vi "Dane.vi"(8 "error in":errorcluster, 9 "Ilość":string, 10 "PIN":string, 11 "Enum":T1(ring)=enum."Deposit") -> (0 "error out":errorcluster, 2 "Konto istniejące":bool=TRUE, 3 "Konto":T2)   [LabVIEW 2021]
doc: "Check if account exist\nReturn info account, account number, first name, last name, amount \nDeposit money and update file.\nWithdraw money and update file"
uses:
  Konto.ctl
  <vilib>/Utility/file.llb/Read Delimited Spreadsheet (string).vi
  <vilib>/Utility/file.llb/Write Delimited Spreadsheet (string).vi
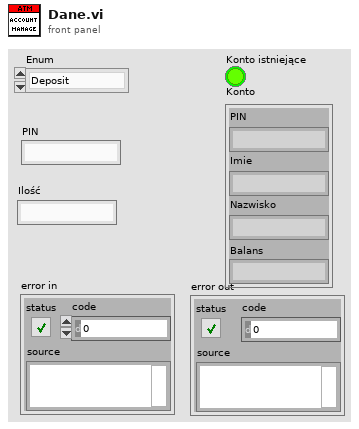
[diagram p1: front panel]
types:
  T1 = enum16{"CheckAccountNumber", "ReturnInfo", "Deposit", "Withdraw"}
  T2 = typedef "Konto.ctl" = cluster{"PIN":string, "Imie":string, "Nazwisko":string, "Balans":string}
  T3 = cluster{"all rows[0]":string, "all rows[1]":string, "all rows[2]":string, "all rows[3]":string}
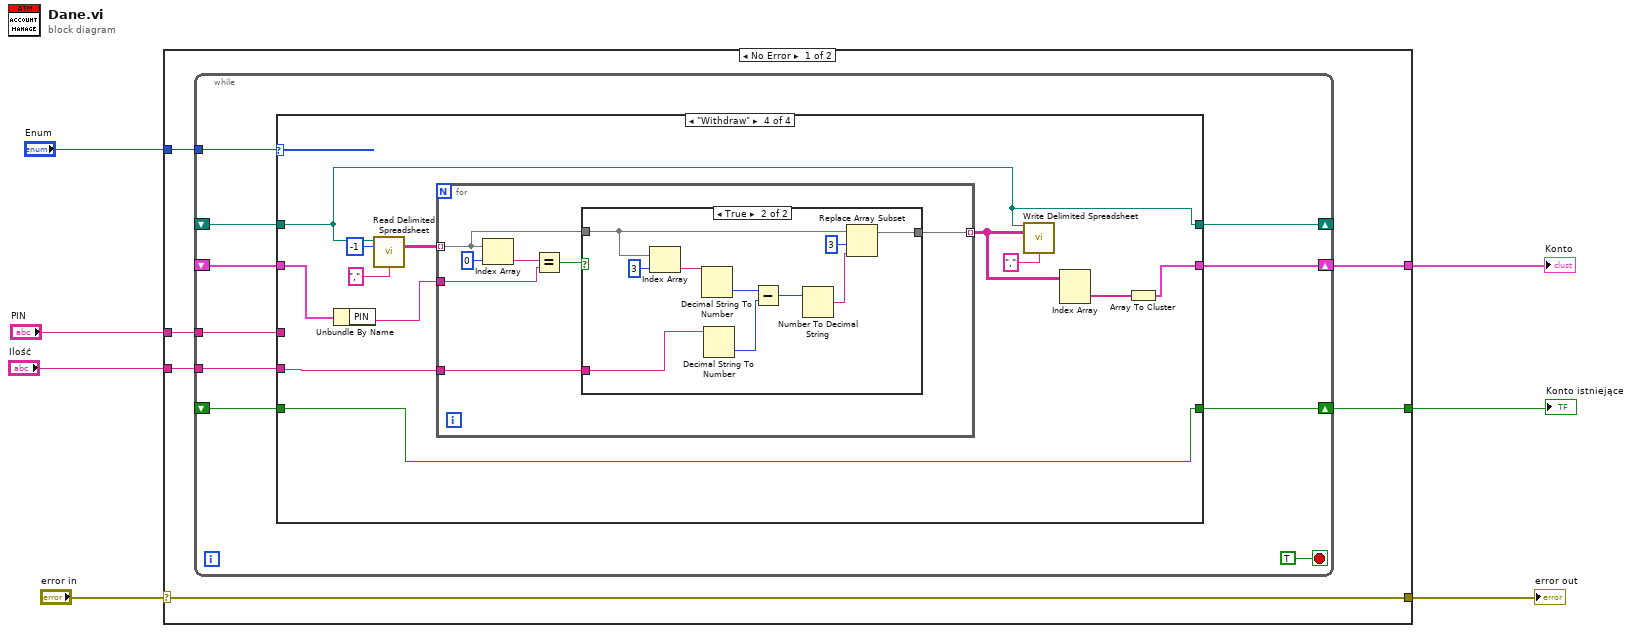
[diagram p0: block diagram]
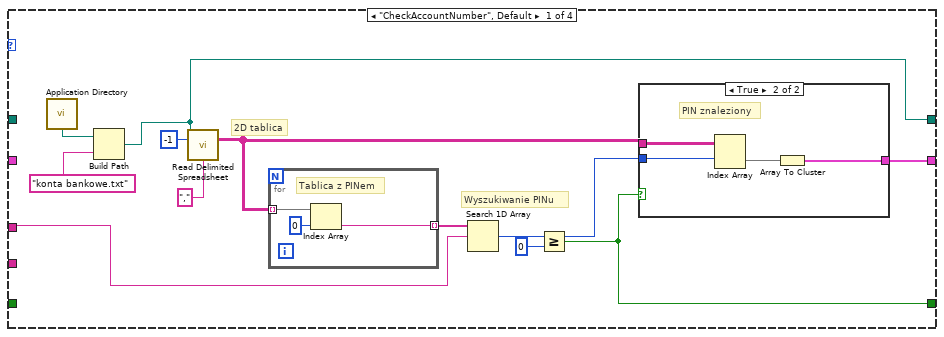
[diagram p2: hidden frame]
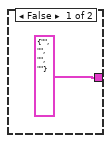
[diagram p3: hidden frame]
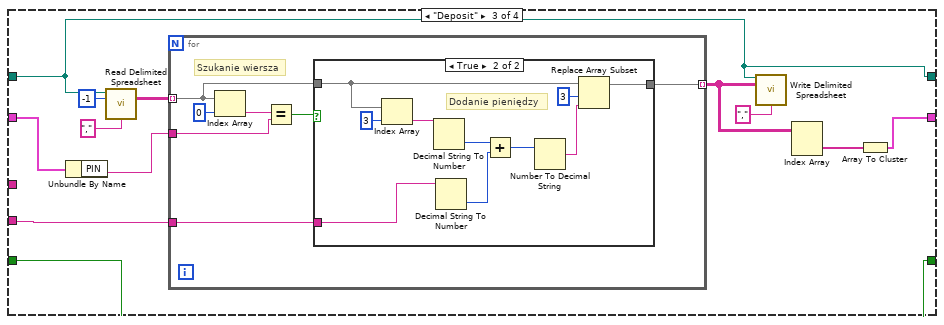
[diagram p5: hidden frame]
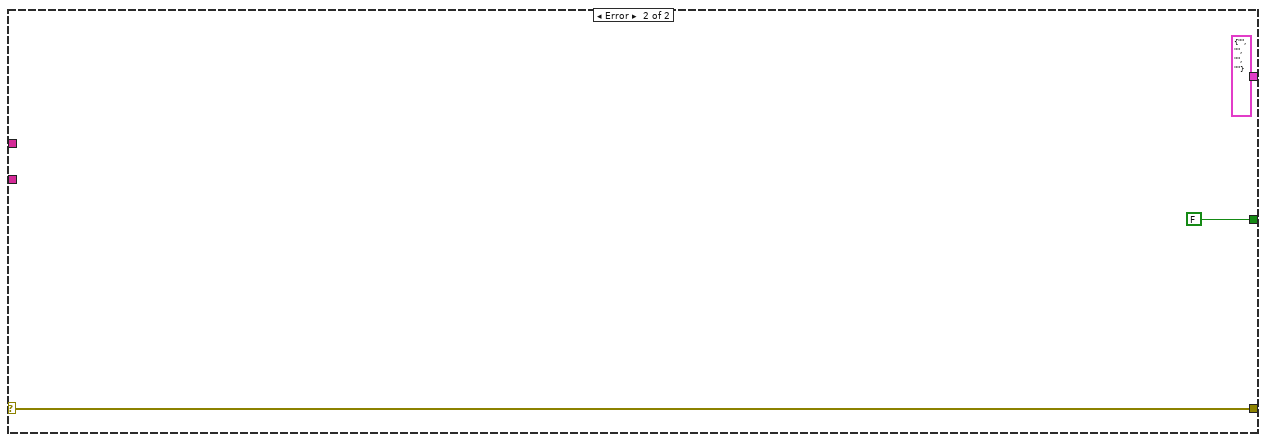
[diagram p8: hidden frame]
diagram:
  n1 = case shown="No Error" "error in" {
    selector: "error in" -> [w12 w109]
    tunnel: "Enum" -> [w13 _]
    tunnel: [w12 w109] -> w5
    tunnel: "PIN" -> [w11 _]
    tunnel: [w10 FALSE] -> w3
    tunnel: [w9 T2 {"PIN"="", "Imie"="", "Nazwisko"="", "Balans"=""} ("Account 2")] -> w2
    tunnel: "Ilość" -> [w8 _]
    frame No Error {
      n2 = while {
        tunnel: w13 -> [w22]
        shift-right: [w21] -> _
        shift-left: _ -> [w15]
        tunnel: w11 -> [w20]
        shift-right: [w19] -> w10
        shift-left: _ -> [w17]
        shift-right: [w18] -> w9
        shift-left: _ -> [w16]
        tunnel: w8 -> [w14]
        stop <- TRUE stop-if-true
        n3 = case shown="\"Withdraw\"" w22 {
          tunnel: [w26 w44 w47 w77] -> w21
          tunnel: w20 -> [w24 _ _ _]
          tunnel: [w28 w46 w48 w78] -> w19
          tunnel: [w27 w45 w49 w79] -> w18
          tunnel: w17 -> [_ w46 w48 w78]
          tunnel: w16 -> [_ w45 w54 w84]
          tunnel: w15 -> [_ w44 w47 w77]
          tunnel: w14 -> [_ _ w53 w83]
          frame "CheckAccountNumber", Default {
            # "2D tablica"
            # "Wyszukiwanie PINu"
            n4 = call <vilib>:"Application Directory.vi"() -> ("Application Directory"=w32:path)
            n5 = Build Path(base path=w32, name or relative path="konta bankowe.txt") -> (appended path=w26:path)
            n6 = call-poly <vilib>:"Read Delimited Spreadsheet.vi"("file path (dialog if empty)"=w26, "number of rows (all:-1)"=-1, "delimiter (\\t)"="," ("delimiter (\\t)")) -> ("all rows"=w25:string[][])  [unwired: 7 in, 5 out]
            n7 = for {
              tunnel: [w42] -> w31 mode=indexing
              tunnel: w25 -> [w41] mode=indexing
              # "Tablica z PINem"
              n8 = Index Array(array=w41, index=0) -> (element=w42:string)
            }
            n9 = Search 1D Array(1D array=w31, element=w24) -> (index of element=w29:i32)  [unwired: 1 in]
            n10 = Greater Or Equal?(x=w29, y=0) -> (x >= y?=w28:bool)
            n11 = case shown="True" w28 {
              tunnel: w25 -> [_ w40]
              tunnel: w29 -> [_ w39]
              tunnel: [T2 {"PIN"="", "Imie"="", "Nazwisko"="", "Balans"=""} ("Account 2") w38] -> w27
              frame False {
              }
              frame True {
                # "PIN znaleziony"
                n12 = Index Array(array=w40, index (row)=w39) -> (element=w37:string[])  [unwired: 1 in]
                n13 = Array To Cluster(array=w37) -> (cluster=w38:T3)
              }
            }
          }
          frame "ReturnInfo" {
          }
          frame "Deposit" {
            n14 = Unbundle By Name(w54) -> ("PIN"=w55:string)
            n15 = call-poly <vilib>:"Read Delimited Spreadsheet.vi"("file path (dialog if empty)"=w47, "number of rows (all:-1)"=-1, "delimiter (\\t)"="," ("delimiter (\\t)")) -> ("all rows"=w56:string[][])  [unwired: 7 in, 5 out]
            n16 = for {
              tunnel: w56 -> [w61] mode=indexing
              tunnel: w55 -> [w63]
              tunnel: w53 -> [w60]
              tunnel: [w59] -> w50 mode=indexing
              # "Szukanie wiersza"
              n17 = Index Array(array=w61, index=0) -> (element=w64:string)
              n18 = Equal?(x=w64, y=w63) -> (x = y?=w62:bool)
              n19 = case shown="True" w62 {
                tunnel: w61 -> [w66 w75]
                tunnel: w60 -> [_ w71]
                tunnel: [w66 w67] -> w59
                frame False {
                }
                frame True {
                  # "Dodanie pieniędzy"
                  n20 = Index Array(array=w75, index=3) -> (element=w73:string)
                  n21 = Decimal String To Number(string=w73) -> (number=w72:i32)  [unwired: 2 in, 1 out]
                  n22 = Decimal String To Number(string=w71) -> (number=w70:i32)  [unwired: 2 in, 1 out]
                  n23 = Add(x=w72, y=w70) -> (x+y=w69:i32)
                  n24 = Number To Decimal String(number=w69) -> (decimal integer string=w68:string)  [unwired: 1 in]
                  n25 = Replace Array Subset(array=w75, new element=w68, index=3) -> (w67:string[])
                }
              }
            }
            n26 = call-poly <vilib>:"Write Delimited Spreadsheet.vi"("file path (dialog if empty)"=w47, "2D data"=w50, "delimiter (\\t)"="," ("delimiter (\\t)")) -> ()  [unwired: 11 in, 2 out]
            n27 = Index Array(array=w50) -> (element=w51:string[])  [unwired: 2 in]
            n28 = Array To Cluster(array=w51) -> (cluster=w49:T3)
          }
          frame "Withdraw" {
            n29 = Unbundle By Name(w84) -> ("PIN"=w85:string)
            n30 = call-poly <vilib>:"Read Delimited Spreadsheet.vi"("file path (dialog if empty)"=w77, "number of rows (all:-1)"=-1, "delimiter (\\t)"="," ("delimiter (\\t)")) -> ("all rows"=w86:string[][])  [unwired: 7 in, 5 out]
            n31 = for {
              tunnel: w86 -> [w91] mode=indexing
              tunnel: w85 -> [w93]
              tunnel: w83 -> [w90]
              tunnel: [w89] -> w80 mode=indexing
              n32 = Index Array(array=w91, index=0) -> (element=w94:string)
              n33 = Equal?(x=w94, y=w93) -> (x = y?=w92:bool)
              n34 = case shown="True" w92 {
                tunnel: w91 -> [w96 w105]
                tunnel: w90 -> [_ w101]
                tunnel: [w96 w97] -> w89
                frame False {
                }
                frame True {
                  n35 = Index Array(array=w105, index=3) -> (element=w103:string)
                  n36 = Decimal String To Number(string=w103) -> (number=w102:i32)  [unwired: 2 in, 1 out]
                  n37 = Decimal String To Number(string=w101) -> (number=w100:i32)  [unwired: 2 in, 1 out]
                  n38 = Subtract(x=w102, y=w100) -> (x-y=w99:i32)
                  n39 = Number To Decimal String(number=w99) -> (decimal integer string=w98:string)  [unwired: 1 in]
                  n40 = Replace Array Subset(array=w105, new element=w98, index=3) -> (w97:string[])
                }
              }
            }
            n41 = call-poly <vilib>:"Write Delimited Spreadsheet.vi"("file path (dialog if empty)"=w77, "2D data"=w80, "delimiter (\\t)"="," ("delimiter (\\t)")) -> ()  [unwired: 11 in, 2 out]
            n42 = Index Array(array=w80) -> (element=w81:string[])  [unwired: 2 in]
            n43 = Array To Cluster(array=w81) -> (cluster=w79:T3)
          }
        }
      }
    }
    frame Error {
    }
  }
  "error out" <- w5
  "Konto istniejące" <- w3
  "Konto" <- w2
